vi "CA Batch.vi"(6 "Select directory with EYE files":path) -> ()   [LabVIEW 2022 SP3]
uses:
  <vilib>/Analysis/baseanly.llb/Mean (DBL).vi
  <vilib>/Utility/file.llb/Read Delimited Spreadsheet (DBL).vi
  <vilib>/Utility/file.llb/Write Delimited Spreadsheet (DBL).vi
  <vilib>/Analysis/NI_AALBase.lvlib
panel:
  in  "Excitation Type":u16(ring) items=["tone burst", "chirp"]
  in  "Save Event Index":bool
  out "event indexes":dbl[](array[numeric])
  in  "Cal Date":enum16{"April 2007", "Jan 2008"}(ring)=enum."Jan 2008"
  out "Therapy Parameters":T1 {"Aamplitude (mV)" min=50 max=1000 format="%.2f"; "Cycles (s)" format="%.3f"; "Theraputic Freq (MHz)" format="%.3f"}
  out "Scatter 20":cluster{dbl[], "Best Linear Fit":dbl[]}[](graph)
  in  "thresh (dB)":dbl=25.0
  in  "Save Stats":bool
  in  "Save Image":bool
  out "Current File":string
  out "?":string
  out "Cluster":T2
  in  "note":string
  in  "File Names":i32[](listbox)
  in  "Use Selected Files":bool
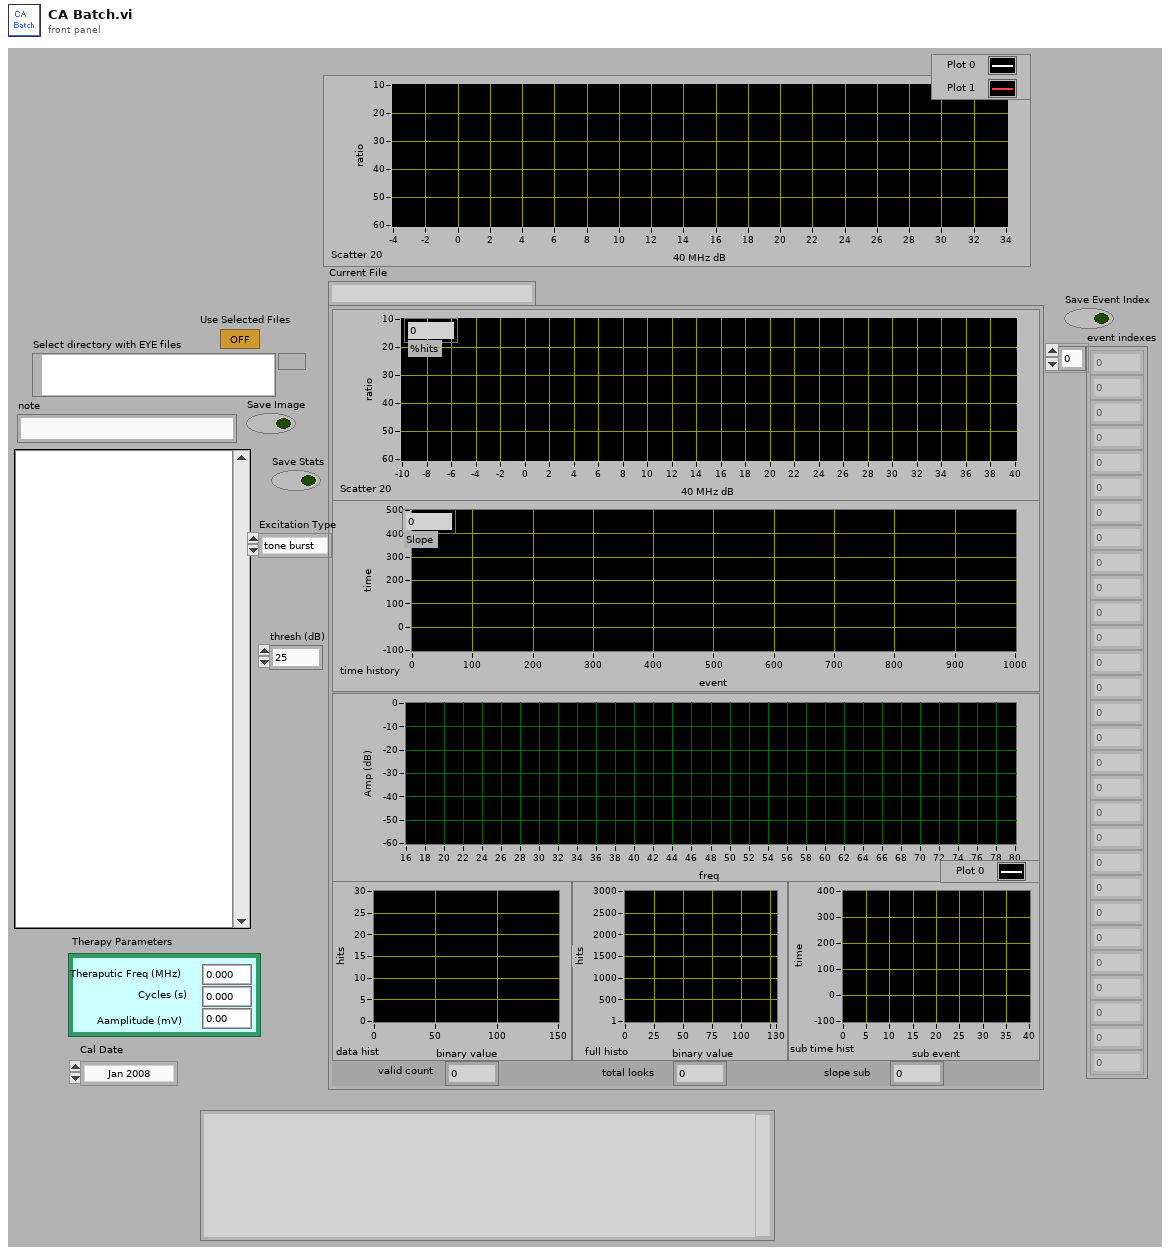
[diagram p1: front panel]
types:
  T1 = cluster{"Theraputic Freq (MHz)":sgl, "Cycles (s)":sgl, "Aamplitude (mV)":sgl, "Lines Before":u16, "Lines After":u16}
  T2 = cluster{"Scatter 20":cluster{dbl[], "Best Linear Fit":dbl[]}[], "time history":cluster{i32[], "Best Linear Fit":dbl[]}[], "spec":cluster{i32, "df":dbl, dbl[][]}, "data hist":cluster{"X Values":dbl[], "Histogram: h(x)":i32[]}, "full histo":cluster{"X Values":dbl[], "Histogram: h(x)":i32[]}, "sub time hist":cluster{i32[], "Best Linear Fit":dbl[]}[], "%hits":dbl, "Slope":dbl, "valid count":i32, "total looks":i32, "slope sub":i32}
  T3 = typedef "Header.ctl" = cluster{"header info":cluster{"Header":string, "Head length":i16}, "A/D info":cluster{"# rf points per line":u16, "# lines per scan":u16, "sample rate MHz":u16, "# A/D bits":i16, "# bytes per A/D":u16, "TGC Flag":u16, "A/D Type":string}, "Tranducer Info":cluster{"bandwidth":sgl, "center freq":sgl, "start freq":sgl, "ID":i32}, "Scan Info":cluster{"delay":sgl, "pivot distance":sgl, "sector scan angle":sgl, "operator":string, "Scan Mode":string, "location":string}, "Time/Date Info":cluster{"date":string, "time":string}, "RF Info":cluster{"RF file name":string, "RF file att":string, "RF cal file name":string, "RF cal file att":string}, "Patient Info":cluster{"ID":string, "extended ID":string, "age":u16, "sex":string, "previously\nscanned":string, "PSA":sgl, "LOS":u8, "Ethnicty 2":u8, "Race":u8}, "Tissue Type":cluster{"organ":i16, "disease type":i16, "disease location":i16, "IQ_pts":u16, "RcvBuffer":u8, "RcvFrame":u16, "IQBuff":u8, "IQFrame":u16, "IQPage":u8}, "Votage scaling":cluster{"Digitizer (dB)":sgl, "Gain (dB)":sgl, "Atten (dB)":sgl}, "Comment":string, "Misc Info":cluster{"avg num":u16, "c speed":i16, "Div By or SF zones":i16, "XMIT CHS":u8, "RCV CHS":u8, "Xmit angle":sgl}, "Therapy Parameters":cluster{"Theraputic Freq (MHz)":sgl, "Time on (s)":sgl, "Therapy amplitude (mV)":sgl, "Lines Before":u16, "Lines After":u16}, "Scan Settings":cluster{"Energy (uJ or V)":u8, "Damp (Ohm) or Fc":u8, "HP Filt (KHz)":u8, "LP Filt (MHz)":u8, "Gain (db)":u8, "prf (kHz)":sgl, "Distance between\nscan lines (um)":u16, "Distance between\nscan planes (um)":u16, "Scan line gap (um)":sgl, "Scan plane gap (um)":sgl}, "Compression Parameters":cluster{"F1 (MHz)":sgl, "F2 (MHz)":sgl, "% taper":sgl, "duration":sgl}, "Patient Info Xtra":cluster{"First Name":string, "Last Name":string, "Notes":string}, "ROI Box":u16[]}
  T4 = cluster{"Theraputic Freq (MHz)":sgl, "Time on (s)":sgl, "Therapy amplitude (mV)":sgl, "Lines Before":u16, "Lines After":u16}
  T5 = cluster{"F1 (MHz)":sgl, "F2 (MHz)":sgl, "% taper":sgl, "duration":sgl}
  T6 = cluster{"Theraputic Freq (MHz)":i32, "Time on (s)":i32, "Therapy amplitude (mV)":i32, "Lines Before":i32, "Lines After":i32}
  T7 = cluster{"40 MHz mean":dbl, "40 MHz SD":dbl, "Ratio Mean":dbl, "Ratio SD":dbl, "Hit frac":dbl, "Hit Num":i32, "slope cum":dbl, "r^2 cum":dbl, "slope sub":dbl, "r^2 sub":dbl}
  T8 = cluster{"X Values":dbl[], "Histogram: h(x)":i32[]}
  T9 = cluster{"Scatter":cluster{dbl[], "Best Linear Fit":dbl[]}[], "total time":cluster{i32[], "Best Linear Fit":dbl[]}[], "Spectra":cluster{i32, "df":dbl, dbl[][]}, "Histogram":cluster{"X Values":dbl[], "Histogram: h(x)":i32[]}, "Histogram":cluster{"X Values":dbl[], "Histogram: h(x)":i32[]}, "sub time":cluster{i32[], "Best Linear Fit":dbl[]}[], "Hit frac":dbl, "slope cum":dbl, "number":i32, "number":i32, "slope sub":dbl}
  T10 = typedef "imagedata.ctl" = cluster{"image type":i32, "image depth":i32, "image":u8[], "mask":u8[], "colors":u32[], "Rectangle":cluster{"left":i16, "top":i16, "right":i16, "bottom":i16}}
  T11 = cluster{"left":i16, "top":i16, "right":i16, "bottom":i16}
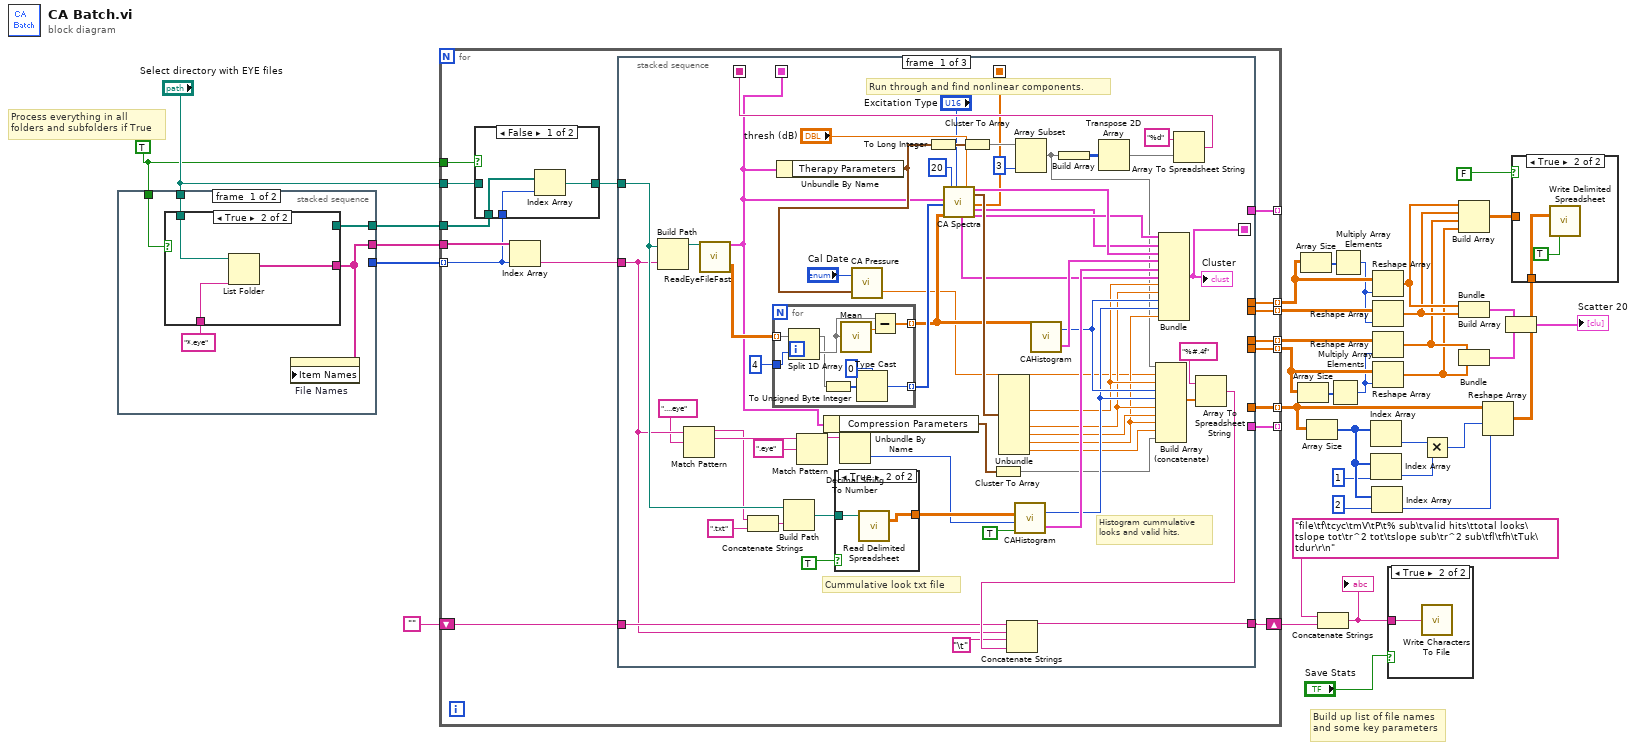
[diagram p0: block diagram]
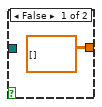
[diagram p5: hidden frame]
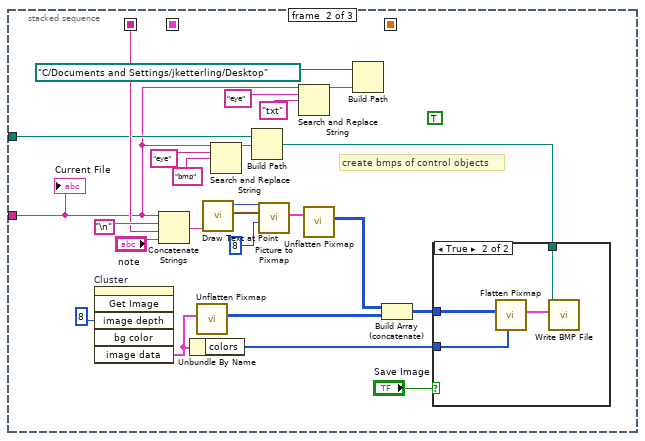
[diagram p6: hidden frame]
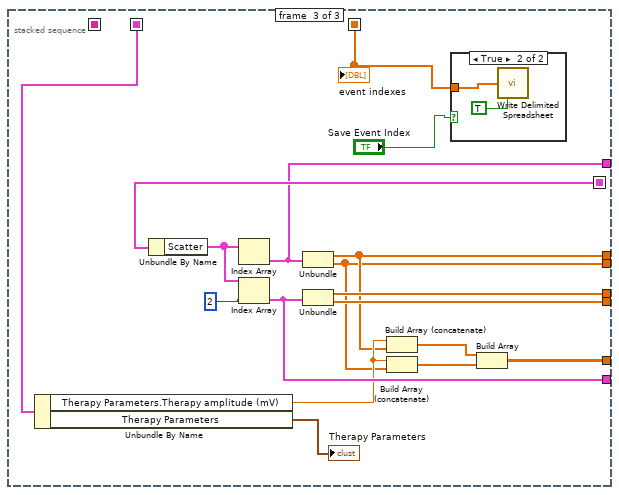
[diagram p8: hidden frame]
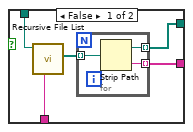
[diagram p10: hidden frame]
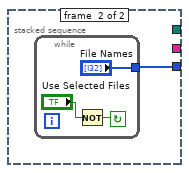
[diagram p11: hidden frame]
diagram:
  w2 = TRUE
  # "Process everything in all folders and subfolders if True"
  # "Build up list of file names and some key parameters"
  n1 = stacked-sequence {
    tunnel: [w41 _] -> w36
    tunnel: "Select directory with EYE files" -> [w40 _]
    tunnel: [_ w53] -> w35
    tunnel: w2 -> [w38 _]
    tunnel: [w37 _] -> w1
    frame #0 {
      n2 = case shown="True" w38 {
        tunnel: [w43 w52] -> w41
        tunnel: w40 -> [w45 w51]
        tunnel: "*.eye" ("pattern") -> [w46 w50]
        tunnel: [w42 _] -> w37
        frame False {
          n3 = call <vilib>:"Recursive File List.vi"("pattern"=w46, "Folder Path"=w45) -> ("All Files in Dir"=w44:path[])  [unwired: 2 in, 7 out]
          n4 = for {
            tunnel: w44 -> [w49] mode=indexing
            tunnel: [w48] -> w43 mode=indexing
            tunnel: [w47] -> w42 mode=indexing
            n5 = Strip Path(path=w49) -> (stripped path=w47:path, name=w48:string)
          }
        }
        frame True {
          n6 = List Folder(path=w51, pattern=w50) -> (filenames=w52:string[])  [unwired: 1 in, 4 out]
        }
      }
      n7 = property on="File Names" class="LstBox (strict)"("Item Names"=w41) -> ()  [unwired: 2 in, 2 out]
    }
    frame #1 {
      n8 = while {
        tunnel: ["File Names"] -> w53
        stop <- w54 continue-if-true
        n9 = Not(x="Use Selected Files") -> (.not. x?=w54:bool)
      }
    }
  }
  n10 = for {
    tunnel: "Select directory with EYE files" -> [w58]
    tunnel: w36 -> [w72]
    tunnel: w35 -> [w61] mode=indexing
    shift-right: [w70] -> w32
    shift-left: "" -> [w71]
    tunnel: [w69] -> w29 mode=indexing
    tunnel: [w68] -> w27 mode=indexing
    tunnel: [w67] -> w25 mode=indexing
    tunnel: [w66] -> w24 mode=indexing
    tunnel: [w65] -> _ mode=indexing
    tunnel: [w64] -> _ mode=indexing
    tunnel: [w63] -> w10 mode=indexing
    tunnel: w2 -> [w62]
    tunnel: w1 -> [w60]
    n11 = case shown="False" w62 {
      tunnel: w61 -> [w75 _]
      tunnel: w60 -> [w74 _]
      tunnel: [w73 w76] -> w59
      tunnel: w58 -> [_ w76]
      frame False {
        n12 = Index Array(array=w74, index=w75) -> (element=w73:path)
      }
      frame True {
      }
    }
    n13 = Index Array(array=w72, index=w61) -> (element=w57:string)
    n14 = stacked-sequence {
      seq-local: [w126 _ _] -> [_ w158 _]
      seq-local: [w108 _ _] -> [_ _ w192]
      seq-local: [w77 _ _] -> [_ _ w179]
      seq-local: [w103 _ _] -> [_ _ w178]
      tunnel: w57 -> [w83 w147 _]
      tunnel: w59 -> [w133 w153 _]
      tunnel: [w109 _ _] -> w70
      tunnel: w71 -> [w110 _ _]
      tunnel: [_ _ w182] -> w69
      tunnel: [_ _ w181] -> w68
      tunnel: [_ _ w187] -> w67
      tunnel: [_ _ w186] -> w66
      tunnel: [_ _ w189] -> w65
      tunnel: [_ _ w188] -> w64
      tunnel: [_ _ w180] -> w63
      frame #0 {
        # "Histogram cummulative looks and valid hits."
        # "Cummulative look txt file"
        # "Run through and find nonlinear components."
        n15 = Build Path(base path=w133, name or relative path=w83) -> (appended path=w134:path)
        n16 = Match Pattern(string=w83, regular expression="....eye") -> (before substring=w84:string, match substring=w85:string)  [unwired: 3 out]
        n17 = call "ReadEyeFileFast.vi"("new file path"=w134) -> ("2-D data array"=w99:sgl[][], "Header In"=w77:T3)  [unwired: 1 in, 16 out]
        n18 = Concatenate Strings(w84, ".txt" ("regular expression")) -> (w89:string)
        n19 = for {
          tunnel: w99 -> [w144] mode=indexing
          tunnel: [w145] -> w98 mode=indexing
          tunnel: 4 -> [w143]
          tunnel: [w138] -> w101 mode=indexing
          n20 = Split 1D Array(array=w144, index=w143) -> (first subarray=w139:sgl[], second subarray=w142:sgl[])
          n21 = To Unsigned Byte Integer(number=w139) -> (unsigned 8bit integer=w141:u8[])
          n22 = call-poly <vilib>:"Mean.vi"("X"=w142) -> ("mean"=w146:dbl)  [unwired: 1 out]
          n23 = Type Cast(type=u32 0, x=w141) -> (*(type *) &x=w138:u32)
          n24 = Subtract(x=w142, y=w146) -> (x-y=w145:dbl[])
        }
        n25 = Unbundle By Name(w77) -> ("Therapy Parameters"=w78:T4)
        n26 = Build Path(base path=w133, name or relative path=w89) -> (appended path=w130:path)
        n27 = Match Pattern(string=w85, regular expression=".eye") -> (before substring=w87:string)  [unwired: 4 out]
        n28 = Unbundle By Name(w77) -> ("Compression Parameters"=w79:T5)
        n29 = case shown="True" TRUE ("Case Constant\n(See Context Help)") {
          tunnel: [sgl[][] [] ("all rows") w136] -> w131
          tunnel: w130 -> [_ w137]
          frame False {
          }
          frame True {
            n30 = call-poly <vilib>:"Read Delimited Spreadsheet.vi"("file path (dialog if empty)"=w137) -> ("all rows"=w136:dbl[][])  [unwired: 9 in, 5 out]
          }
        }
        n31 = Decimal String To Number(string=w87) -> (number=w88:i32)  [unwired: 3 out]
        n32 = call "CA Pressure.vi"("Therapy Parameters"=w78, "Cal Date"="Cal Date") -> ("p (MPa)"=w92:dbl)  [unwired: 1 out]
        n33 = To Long Integer(number=w78) -> (32bit integer=w129:T6)
        n34 = call "CA Spectra.vi"("Header In"=w77, "time array"=w101, "Data in"=w98, "2nd freq"=20, "Excitation Type"="Excitation Type", "sub thresh"="thresh (dB)") -> ("sub time"=w100:cluster{i32[], "Best Linear Fit":dbl[]}[], "Spectra"=w116:cluster{i32, "df":dbl, dbl[][]}, "output params"=w107:T7, "Sub indexes"=w103:dbl[], "total time"=w102:cluster{i32[], "Best Linear Fit":dbl[]}[], "Scatter"=w105:cluster{dbl[], "Best Linear Fit":dbl[]}[])  [unwired: 4 in, 4 out]
        n35 = Cluster To Array(cluster=w129) -> (array=w128:i32[])
        n36 = Cluster To Array(cluster=w79) -> (array=w80:sgl[])
        n37 = Unbundle(w107) -> ("Hit frac"=w104:dbl, "slope cum"=w95:dbl, "r^2 cum"=w97:dbl, "slope sub"=w94:dbl, "r^2 sub"=w96:dbl)  [unwired: 5 out]
        n38 = call "CAHistogram.vi"("Peak File?"=TRUE, "index"=w88, "all rows"=w131) -> ("Histogram"=w120:T8, "number"=w114:i32)  [unwired: 1 in]
        n39 = Array Subset(array=w128, length=3) -> (w93:i32[])  [unwired: 1 in]
        n40 = call "CAHistogram.vi"("Data"=w98) -> ("Histogram"=w121:T8, "number"=w115:i32)  [unwired: 3 in]
        n41 = Build Array(w93) -> (w124:i32[][])
        n42 = Transpose 2D Array(2D array=w124) -> (transposed array=w123:i32[][])
        n43 = Build Array (concatenate)(w93, w92, w104, w115, w114, w95, w97, w94, w96, w80) -> (w118:dbl[])
        n44 = Bundle("Scatter"=w105, "total time"=w102, "Spectra"=w116, "Histogram"=w121, "Histogram"=w120, "sub time"=w100, "Hit frac"=w104, "slope cum"=w95, "number"=w115, "number"=w114, "slope sub"=w94) -> (w108:T9)  [unwired: 1 out]
        "Cluster" <- w108
        n45 = Array To Spreadsheet String(array=w123, 3:"%d" ("format string")) -> (spreadsheet string=w126:string)  [unwired: 1 out]
        n46 = Array To Spreadsheet String(array=w118, 3:"%#.4f" ("format string")) -> (spreadsheet string=w112:string)  [unwired: 1 out]
        n47 = Concatenate Strings(w110, w83, "\t", w112) -> (w109:string)
      }
      frame #1 {
        (unwired) TRUE
        # "create bmps of control objects"
        n48 = invoke on="Cluster" class="Clust (strict)" method="Get Image"("image depth"=8) -> ("image data"=w155:T10)  [unwired: 5 in, 5 out]
        n49 = Concatenate Strings(w147, "\n", w158, "note") -> (w165:string)
        n50 = Unbundle By Name(w155) -> ("colors"=w171:u32[])
        n51 = call <vilib>:"Unflatten Pixmap.vi"("image data"=w155) -> ("8-bit pixmap"=w156:u8[][])  [unwired: 10 out]
        n52 = call <vilib>:"Draw Text at Point.vi"("text"=w165) -> ("text rect"=w164:T11, "new picture"=w160:picture)  [unwired: 8 in, 1 out]
        n53 = Search and Replace String(input string=w147, search string="eye", replace string="bmp") -> (result string=w149:string)  [unwired: 1 in, 7 out]
        n54 = Build Path(base path=w153, name or relative path=w149) -> (appended path=w168:path)
        n55 = call <vilib>:"Picture to Pixmap.vi"("depth"=8, "rect"=w164, "picture"=w160) -> ("image data"=w163:T10)  [unwired: 1 in, 7 out]
        n56 = Search and Replace String(input string=w147, search string="eye", replace string="txt") -> (result string=w148:string)  [unwired: 1 in, 7 out]
        n57 = call <vilib>:"Unflatten Pixmap.vi"("image data"=w163) -> ("8-bit pixmap"=w162:u8[][])  [unwired: 10 out]
        n58 = Build Path(base path=path "C:/Documents and Settings/jketterling/Desktop", name or relative path=w148) -> ()  [unwired: 1 out]
        n59 = Build Array (concatenate)(w162, w156) -> (w167:u8[][])
        n60 = case shown="True" "Save Image" {
          tunnel: w171 -> [_ w175]
          tunnel: w168 -> [_ w174]
          tunnel: w167 -> [_ w173]
          frame False {
          }
          frame True {
            n61 = call <vilib>:"Flatten Pixmap.vi"("colors"=w175, "8-bit pixmap"=w173) -> ("image data"=w172:T10)  [unwired: 4 in, 5 out]
            n62 = call <vilib>:"Write BMP File.vi"("image data"=w172, "path to BMP file"=w174) -> ()  [unwired: 1 in, 9 out]
          }
        }
        "Current File" <- w147
      }
      frame #2 {
        n63 = Unbundle By Name(w179) -> ("Therapy Parameters.Therapy amplitude (mV)"=w185:sgl, "Therapy Parameters"=→"Therapy Parameters":T4)
        n64 = Unbundle By Name(w192) -> ("Scatter"=w191:cluster{dbl[], "Best Linear Fit":dbl[]}[])
        n65 = Index Array(array=w191) -> (element=w189:cluster{dbl[], "Best Linear Fit":dbl[]})  [unwired: 1 in]
        n66 = Index Array(array=w191, index=2) -> (element=w188:cluster{dbl[], "Best Linear Fit":dbl[]})
        n67 = Unbundle(w189) -> (w182:dbl[], "Best Linear Fit"=w181:dbl[])
        n68 = Unbundle(w188) -> (w187:dbl[], "Best Linear Fit"=w186:dbl[])
        n69 = Build Array (concatenate)(w185, w182) -> (w183:dbl[])
        n70 = Build Array (concatenate)(w185, w181) -> (w184:dbl[])
        n71 = case shown="True" "Save Event Index" {
          tunnel: w178 -> [_ w194]
          frame False {
          }
          frame True {
            n72 = call-poly <vilib>:"Write Delimited Spreadsheet.vi"("1D data"=w194, "transpose? (no:F)"=TRUE) -> ()  [unwired: 12 in, 2 out]
          }
        }
        n73 = Build Array(w183, w184) -> (w180:dbl[][])
        "event indexes" <- w178
      }
    }
  }
  n74 = Array Size(array=w24) -> (size(s)=w26:i32[])
  n75 = Array Size(array=w29) -> (size(s)=w28:i32[])
  n76 = Array Size(array=w10) -> (size(s)=w13:i32[])
  n77 = Concatenate Strings("file\tf\tcyc\tmV\tP\t% sub\tvalid hits\ttotal looks\tslope tot\tr^2 tot\tslope sub\tr^2 sub\tfl\tfh\tTuk\tdur\r\n", w32) -> (w31:string)
  "?" <- w31
  n78 = Multiply Array Elements(1:w26) -> (0:w23:i32)
  n79 = Multiply Array Elements(1:w28) -> (0:w22:i32)
  n80 = Index Array(array=w13) -> (element=w9:i32)  [unwired: 1 in]
  n81 = Index Array(array=w13, index=1) -> (element=w7:i32)
  n82 = Index Array(array=w13, index=2) -> (element=w6:i32)
  n83 = Reshape Array(w29, w22) -> (w19:dbl[])
  n84 = Reshape Array(w27, w22) -> (w18:dbl[])
  n85 = Reshape Array(w25, w23) -> (w17:dbl[])
  n86 = Reshape Array(w24, w23) -> (w16:dbl[])
  n87 = case shown="True" "Save Stats" {
    tunnel: w31 -> [_ w195]
    frame False {
    }
    frame True {
      n88 = call <vilib>:"Write Characters To File.vi"("character string"=w195) -> ()  [unwired: 2 in, 3 out]
    }
  }
  n89 = Multiply(x=w9, y=w7) -> (x*y=w5:i32)
  n90 = Build Array(w19, w18, w17, w16) -> (w15:dbl[][])
  n91 = Bundle(w19, "Best Linear Fit"=w18) -> (w20:cluster{dbl[], "Best Linear Fit":dbl[]})  [unwired: 1 out]
  n92 = Bundle(w17, "Best Linear Fit"=w16) -> (w21:cluster{dbl[], "Best Linear Fit":dbl[]})  [unwired: 1 out]
  n93 = Reshape Array(w10, w5, w6) -> (w4:dbl[][])
  n94 = Build Array(w20, w21) -> (→"Scatter 20":cluster{dbl[], "Best Linear Fit":dbl[]}[])
  n95 = case shown="True" FALSE ("Case Constant\n(See Context Help) 2") {
    tunnel: w15 -> [_ _]
    tunnel: w4 -> [_ w196]
    frame False {
    }
    frame True {
      n96 = call-poly <vilib>:"Write Delimited Spreadsheet.vi"("2D data"=w196, "transpose? (no:F)"=TRUE) -> ()  [unwired: 12 in, 2 out]
    }
  }
